vi "PRBS64 Parallel Rx - 8 Lanes.vi"(7 "reset":bool, 9 "input valid":bool=TRUE, 11 "rx prbs":u64[](array[numeric])=[0, 0, 0, 0, 0, 0, 0, 0]) -> (1 "output valid":bool, 3 "pattern mismatch":bool)   [LabVIEW 2023, in "Aurora64b66b Utilities FPGA.lvlib"]
uses:
  Aurora64b66b Utilities FPGA.lvlib
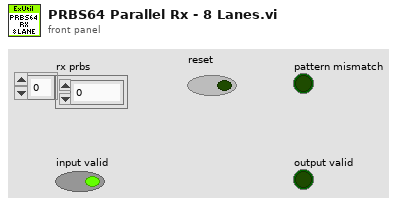
[diagram p1: front panel]
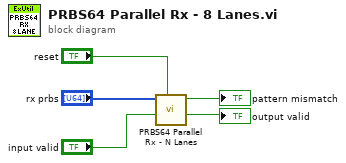
[diagram p0: block diagram]
diagram:
  n1 = call "PRBS64 Parallel Rx - N Lanes.vi"("reset"="reset", "input valid"="input valid", "rx prbs"="rx prbs") -> ("output valid"=→"output valid":bool, "pattern mismatch"=→"pattern mismatch":bool)  [unwired: 7 in]
